vi "GetNumberOfLoops.vi"(8 "error in":errorcluster, 11 "VISA resource name":refnum<visa-resource-name>) -> (0 "error out":errorcluster, 1 "Number of loops":i32, 2 "Number of loops string":string, 3 "VISA resource name out":refnum<visa-resource-name>)   [LabVIEW 2023, in "Thermotron 8800.lvlib"]
doc: "NUML\nCommand name: Send number of loops\nCommand type: Program status\nDescription: Queries the 8800 for the programmed number of loops assigned to the current loop. For nested looping, the value is for the inside loop. The 8800 sends an integer indicating the number of loops assigned to the current loop.\nSyntax: NUML?\nData type: Integer\nQuery example: NUML?\n8800 response: 15 (The number of loops assigned to the current loop is 15.)"
uses:
  Thermotron 8800.lvlib
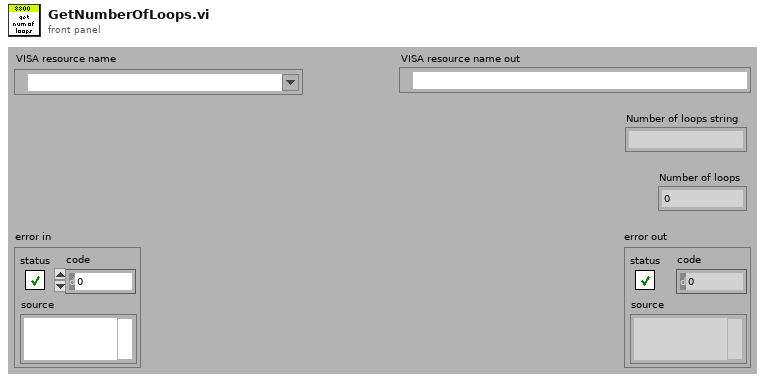
[diagram p1: front panel]
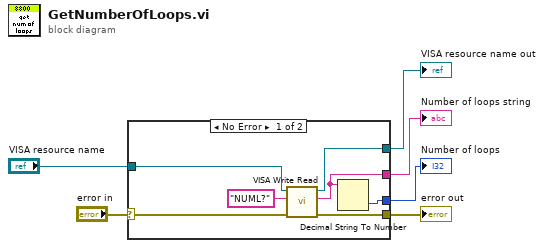
[diagram p0: block diagram]
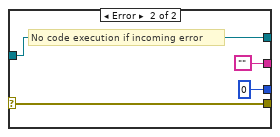
[diagram p2: hidden frame]
diagram:
  n1 = case shown="No Error" "error in" {
    selector: "error in" -> [w13 w17]
    tunnel: [w12 w17] -> w5
    tunnel: "VISA resource name" -> [w11 w14]
    tunnel: [w10 w14] -> w3
    tunnel: [w9 ""] -> w1
    tunnel: [w8 0] -> w2
    frame No Error {
      n2 = call "VISA Write Read.vi"("error in (no error)"=w13, "8800 Command"="NUML?", "VISA Refnum in"=w11) -> ("error out"=w12:errorcluster, "read buffer"=w9:string, "VISA Refnum out"=w10:refnum<visa-resource-name>)  [unwired: 6 in]
      n3 = Decimal String To Number(string=w9) -> (number=w8:i32)  [unwired: 2 in, 1 out]
    }
    frame Error {
      # "No code execution if incoming error"
    }
  }
  "error out" <- w5
  "VISA resource name out" <- w3
  "Number of loops" <- w2
  "Number of loops string" <- w1
